vi "DidInit.vi"(7 "Init?":bool, 8 "error in (no error)":errorcluster, 11 "ModuleAdmin":refnum<class "ModuleAdmin.lvclass">) -> (0 "error out":errorcluster)   [LabVIEW 2014, in "SamplerModule.lvlib"]
uses:
  SamplerModule.lvlib
  <userlib>/NIST/ModuleAdminLib/ModuleAdmin/ModuleAdmin.lvclass
  PublicAPI/Arguments/Broadcasts/clDidInit.ctl
  clEventType.ctl
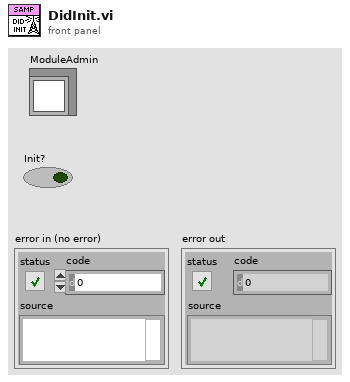
[diagram p1: front panel]
types:
  T1 = typedef "SamplerModule.lvlib/clEventType.ctl" = cluster{"ModuleID":i32, "Data":variant}
  T2 = typedef "SamplerModule.lvlib/clDidInit.ctl" = cluster{"Init?":bool, "ModuleAdmin":refnum<class "ModuleAdmin.lvclass">}
  T3 = typedef "SamplerModule.lvlib/clBroadcastEvents.ctl" = cluster{"DidInit":refnum<user-event>, "StatusUpdate":refnum<user-event>, "ErrorReport":refnum<user-event>, "DidStop":refnum<user-event>, "PathToINI":refnum<user-event>, "GetReading":refnum<user-event>, "IsOverRange":refnum<user-event>, "GetMultiPointReading":refnum<user-event>}
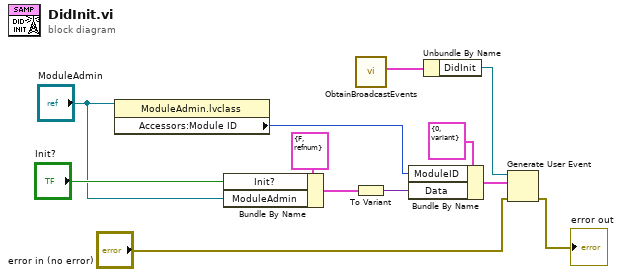
[diagram p0: block diagram]
diagram:
  n1 = property class="ModuleAdmin.lvclass"(reference="ModuleAdmin") -> ("Accessors:Module ID"=w2:i32)  [unwired: 1 in, 2 out]
  n2 = Bundle By Name(cluster=T2 {"Init?"=FALSE, "ModuleAdmin"=refnum} ("clDidInit"), "Init?"="Init?", "ModuleAdmin"="ModuleAdmin") -> (w10:T2)
  n3 = call "ObtainBroadcastEvents.vi"() -> ("SamplerBroadcast"=w11:T3)  [unwired: 10 in, 1 out]
  n4 = To Variant(anything=w10) -> (Variant=w7:variant)
  n5 = Bundle By Name(cluster=T1 {"ModuleID"=0, "Data"=variant} ("clBroadcast"), "ModuleID"=w2, "Data"=w7) -> (w6:T1)
  n6 = Unbundle By Name(w11) -> ("DidInit"=w9:refnum<user-event>)
  n7 = Generate User Event(user event=w9, event data cluster=w6, error in="error in (no error)") -> (error out=→"error out":errorcluster)  [unwired: 1 in, 1 out]
